vi "Merge.vi"(7 "Target Tree ID":string, 8 "Error In":errorcluster, 10 "Source Tree ID":string, 11 "Tree Manager":refnum<data-value>) -> (0 "Error Out":errorcluster, 3 "Tree Manager":refnum<data-value>)   [LabVIEW 2017, in "Tree API.lvlib" / "Tree.lvclass"]
doc: "Merges a source Tree with target Tree. The target Tree ID is the ID used after the merge and the source Tree ID becomes invalid. The merge operation moves all Children and attributes of the source Tree under the target Tree. Both Tree ID have to be valid."
uses:
  Tree.lvclass
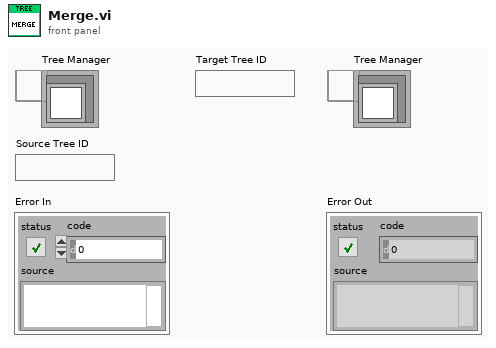
[diagram p1: front panel]
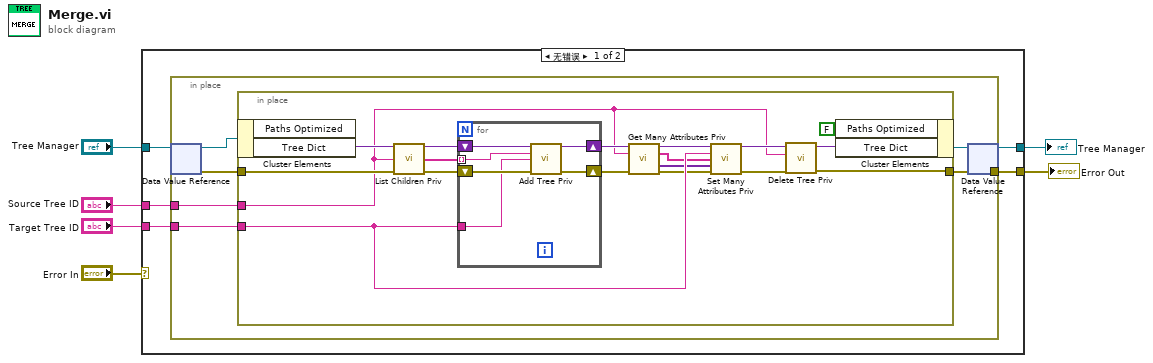
[diagram p0: block diagram]
diagram:
  n1 = case shown="无错误" "Error In" {
    selector: "Error In" -> [_ w42]
    tunnel: "Tree Manager" -> [w11 w43]
    tunnel: [w10 w43] -> w5
    tunnel: [w7 w42] -> w3
    tunnel: "Target Tree ID" -> [w9 _]
    tunnel: "Source Tree ID" -> [w8 _]
    frame No Error {
      n2 = in-place {
        in-place-border: w9 -> [w14]
        in-place-border: w8 -> [w13]
        in-place-border: [w12] -> w7
        n3 = in-place-dvr #1(w11) -> (w17:refnum<class "Tree.lvclass">, w15:errorcluster)
        n4 = in-place {
          in-place-border: w15 -> [w33]
          in-place-border: w14 -> [w27]
          in-place-border: w13 -> [w22]
          in-place-border: [w20] -> w12
          n5 = in-place-cluster #2(w17) -> ("Tree Dict"=w35:variant)  [unwired: 1 out]
          n6 = call "List Children Priv.vi"("Tree Dictionary"=w35, "Parent ID"=w22, "Error In"=w33) -> ("Tree Dictionary Out"=w34:variant, "Child IDs"=w31:string[], "Error Out"=w32:errorcluster)  [unwired: 10 in]
          n7 = for {
            shift-right: [w40] -> w30
            shift-left: w34 -> [w41]
            shift-right: [w36] -> w29
            shift-left: w32 -> [w39]
            tunnel: w27 -> [w37]
            tunnel: w31 -> [w38] mode=indexing
            n8 = call "Add Tree Priv.vi"("Tree Dictionary In"=w41, "Unique ID"=w38, "Parent ID"=w37, "Error In"=w39) -> ("Tree Dictionary Out"=w40:variant, "Error Out"=w36:errorcluster)  [unwired: 10 in]
          }
          n9 = call "Get Many Attributes Priv.vi"("Tree Dictionary In"=w30, "Unique ID"=w22, "error in"=w29) -> ("Tree Dictionary Out"=w28:variant, "Attribute Names"=w19:string[], "Attribute Values"=w26:variant[], "error out"=w25:errorcluster)  [unwired: 7 in, 2 out]
          n10 = call "Set Many Attributes Priv.vi"("Tree Dictionary Out"=w28, "Unique ID"=w27, "Name"=w19, "Data"=w26, "error in"=w25) -> ("Tree Dictionary Out"=w24:variant, "error out"=w23:errorcluster)  [unwired: 8 in, 1 out]
          n11 = call "Delete Tree Priv.vi"("Error In"=w23, "Unique ID"=w22, "Tree Dictionary In"=w24) -> ("Error Out"=w20:errorcluster, "Tree Dictionary Out"=w21:variant)  [unwired: 7 in]
          n12 = in-place-cluster #2("Paths Optimized"=FALSE, "Tree Dict"=w21) -> (w16:refnum<class "Tree.lvclass">)
        }
        n13 = in-place-dvr #1(w16) -> (w10:refnum<data-value>)  [unwired: 1 out]
      }
    }
    frame Error {
    }
  }
  "Tree Manager" <- w5
  "Error Out" <- w3
